vi "Set Ending Tangent.vi"(10 "waypoints":cluster{dbl, dbl}[](array[cluster]), 11 "ending orientation":dbl=nan) -> (3 "ending tangent":cluster{dbl, dbl})   [LabVIEW 2019]
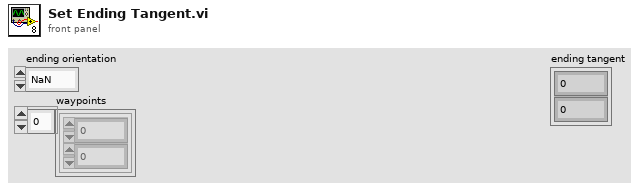
[diagram p1: front panel]
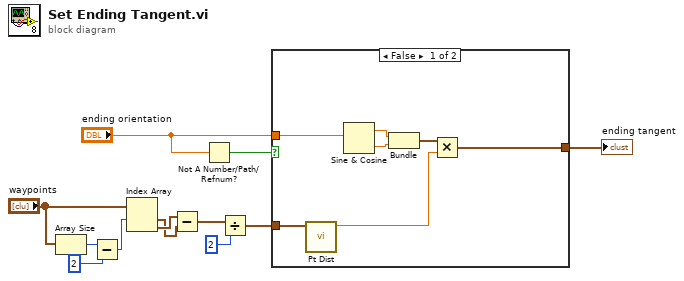
[diagram p0: block diagram]
diagram:
  n1 = Array Size(array="waypoints") -> (size(s)=w9:i32)
  n2 = Subtract(x=w9, y=2) -> (x-y=w7:i32)
  n3 = Index Array(array="waypoints", index #1=w7) -> (element #1=w5:cluster{dbl, dbl}, element #2=w6:cluster{dbl, dbl})  [unwired: 1 in]
  n4 = Subtract(x=w6, y=w5) -> (x-y=w2:cluster{dbl, dbl})
  n5 = Not A Number/Path/Refnum?(number/path/refnum="ending orientation") -> (NaN/Path/Refnum?=w12:bool)
  n6 = Divide(x=w2, y=2) -> (x/y=w1:cluster{dbl, dbl})
  n7 = case shown="False" w12 {
    tunnel: "ending orientation" -> [w19 _]
    tunnel: [w13 w20] -> w4
    tunnel: w1 -> [w15 w20]
    frame False {
      n8 = call "Pt Dist.vi"("point a"=w15) -> ("dist"=w14:dbl)  [unwired: 10 in]
      n9 = Sine & Cosine(0:w19) -> (1:w18:dbl, 2:w17:dbl)
      n10 = Bundle(w18, w17) -> (w16:cluster{dbl, dbl})  [unwired: 1 in]
      n11 = Multiply(x=w16, y=w14) -> (x*y=w13:cluster{dbl, dbl})
    }
    frame True {
    }
  }
  "ending tangent" <- w4
